vi "Serial Loopback DMA (Host).vi"() -> ()   [LabVIEW 2012]
doc: "This is the top level VI for a cRIO target. This example will perform a read and a write from the same port on the 987x module. You can use this VI to verify that the port is working correctly. It uses two DMA channels for communication, one channel from the FPGA to the controller and one channel from the controller to the FPGA. For this reason a cRIO-900x contoller can not be used with this VI. You must use the other examples in this program as they only use DMA from the FPGA to the controller, which is supported by all cRIO controllers.\n\nPlease see the block diagram for more detailed comments."
uses:
  <vilib>/FPGAPlugInAG/cRIO-9113/niLvFpga_Open_cRIO-9113.vi
  <vilib>/FPGAPlugInAG/cRIO-9113/niLvFpga_Reset_cRIO-9113.vi
  <vilib>/FPGAPlugInAG/cRIO-9113/niLvFpga_Run_cRIO-9113.vi
  <vilib>/Utility/error.llb/Error Cluster From Error Code.vi
  <vilib>/RVI Host/nirviSupport.llb/nirviErrorClusterFromErrorCode.vi
  <vilib>/rvi/errors/niLvFpgaAdjustHostInterfaceError.vi
  <vilib>/FPGAPlugInAG/cRIO-9113/niLvFpga_Close_cRIO-9113.vi
  <vilib>/rvi/interface/nirviOpenFPGA/nirviOpenFPGA.xnode
  Program Files (x86)/National Instruments/LabVIEW 2012/examples/CompactRIO/Module Specific/NI 987x/Serial Loopback/FPGA Bitfiles/NI-987xSerialLoo_FPGATarget4_9870InterfaceDMA_lMxNdb7MvEs.lvbitx
  Program Files (x86)/National Instruments/LabVIEW 2012/examples/CompactRIO/Module Specific/NI 987x/Serial Loopback/VIs/9870 Interface DMA (FPGA).vi
  <vilib>/rvi/interface/nirviMethod/nirviMethod.xnode
  <vilib>/rvi/interface/nirviCloseFPGA/nirviCloseFPGA.xnode
  901x DMA FPGA Reference.ctl
  <vilib>/rvi/interface/nirviMethod/StockFPGA_InlinedMethodWaitForSingleIRQ.vi
  <vilib>/FPGAPlugInAG/cRIO-9113/niLvFpga_WaitOnIrq_cRIO-9113.vi
panel:
  out "Byte Count":u32
  in  "Byte Timeout":i32=500
  in  "Bytes to Read":i32=64
  out "Bytes Received":u32
  out "Receive String":string
  in  "Send String":string="ABCDEFGHIJKLMNOPQRSTUVWXYZ-abcdefghijklmnopqrstuvwxyz-0123456789"
  # "Transmit"
  # "Receive"
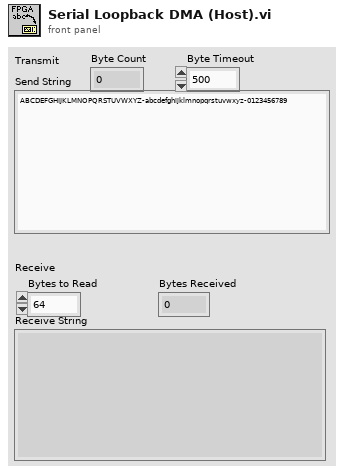
[diagram p1: front panel]
types:
  T1 = typedef "901x DMA FPGA Reference.ctl" = refnum<k20>
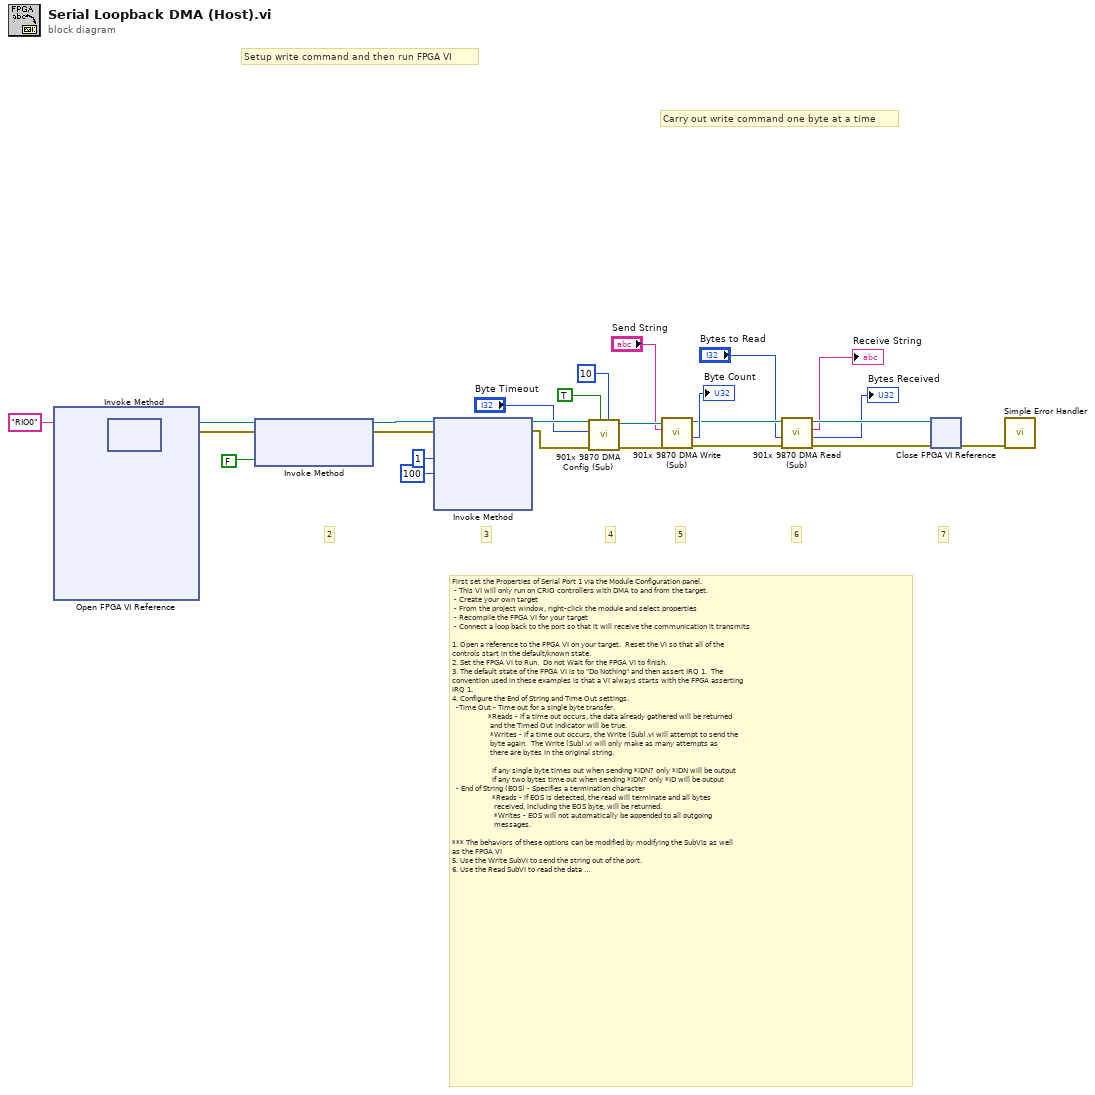
[diagram p0: block diagram]
diagram:
  # "7"
  # "6"
  # "5"
  # "4"
  # "3"
  # "2"
  # "1"
  # "First set the Properties of Serial Port 1 via the Module Configuration panel.\n - This VI will only run on CRIO controllers with DMA to and from the target.\n - Create your own target\n - From the project window, right-click the module and select properties\n - Recompile the FPGA VI for your target\n - Connect a loop back to the port so that it will receive the communication it transmits\n\n1. Open a reference to the FPGA VI on your target.  Reset the VI so that all of the \ncontrols start in the default/known state.\n2. Set the FPGA VI to Run.  Do not Wait for the FPGA VI to finish.\n3. The default state of the FPGA VI is to \"Do Nothing\" and then assert IRQ 1.  The \nconvention used in these examples is that a VI always starts with the FPGA asserting\nIRQ 1.\n4. Configure the End of String and Time Out settings.  \n  -Time Out - Time out for a single byte transfer.\n                  *Reads - if a time out occurs, the data already gathered will be returned\n                   and the Timed Out indicator will be true.\n                   *Writes - if a time out occurs, the Write (Sub).vi will attempt to send the \n                   byte again.  The Write (Sub).vi will only make as many attempts as \n                   there are bytes in the original string.\n                   \n                    If any single byte times out when sending *IDN? only *IDN will be output\n                    If any two bytes time out when sending *IDN? only *ID will be output\n  - End of String (EOS) - Specifies a termination character\n                    *Reads - if EOS is detected, the read will terminate and all bytes \n                     received, including the EOS byte, will be returned.\n                     *Writes - EOS will not automatically be appended to all outgoing \n                     messages.  \n\n*** The behaviors of these options can be modified by modifying the SubVIs as well\nas the FPGA VI\n5. Use the Write SubVI to send the string out of the port.\n6. Use the Read SubVI to read the data returned to the port.\n7. Close the FPGA VI reference and report any errors"
  # "Carry out write command one byte at a time"
  # "Setup write command and then run FPGA VI"
  n1 = xnode "Open FPGA VI Reference"("resource name"="RIO0") -> ("FPGA VI Reference Out"=w23:refnum<k20>, "error out"=w27:errorcluster)  [unwired: 1 in]
  n2 = xnode "Invoke Method"("FPGA VI Reference In"=w23, "error in"=w27) -> ("FPGA VI Reference Out"=w22:refnum<k20>, "error out"=w25:errorcluster)
  n3 = xnode "Invoke Method"("FPGA VI Reference In"=w22, "error in"=w25, "Wait Until Done (F)"=FALSE) -> ("FPGA VI Reference Out"=w20:refnum<k20>, "error out"=w17:errorcluster)
  n4 = xnode "Invoke Method"("FPGA VI Reference In"=w20, "error in"=w17, "IRQ Number(s)"=1, "Timeout (ms)"=100) -> ("FPGA VI Reference Out"=w16:refnum<k20>, "error out"=w15:errorcluster)  [unwired: 2 out]
  n5 = call "901x 9870 DMA Config (Sub).vi"("EOS Byte"=u8 10, "Enable EOS"=TRUE, "error in"=w15, "Byte Timeout"="Byte Timeout", "FPGA In"=w16) -> ("error out"=w11:errorcluster, "FPGA Out"=w10:T1)  [unwired: 5 in]
  n6 = call "901x 9870 DMA Write (Sub).vi"("error in"=w11, "Send Data"="Send String", "FPGA In"=w10) -> ("error out"=w6:errorcluster, "Byte Count"=→"Byte Count":u32, "FPGA Out"=w7:T1)  [unwired: 4 in, 2 out]
  n7 = call "901x 9870 DMA Read (Sub).vi"("error in"=w6, "Number of bytes"="Bytes to Read", "FPGA In"=w7) -> ("error out"=w4:errorcluster, "Byte Count"=→"Bytes Received":u32, "Read Bytes"=→"Receive String":string, "FPGA Out"=w3:T1)  [unwired: 3 in, 2 out]
  n8 = xnode "Close FPGA VI Reference"("FPGA VI Reference In"=w3, "error in"=w4) -> ("error out"=w24:errorcluster)
  n9 = call <vilib>:"Simple Error Handler.vi"("error in (no error)"=w24) -> ()  [unwired: 1 in, 8 out]
